vi "Configure FRTD.vi"(0 "VISA resource name":refnum<visa-resource-name>, 1 "FRTD Type (0: PT100)":u16(ring) items=["PT100", "D100", "F100", "PT3916", "PT385", "USER"], 5 "error in (no error)":errorcluster, 6 "Scan List (Empty)":string, 7 "R Zero (100)":i32=100, 9 "Alpha (0.00385)":dbl=0.00385, 11 "Beta (0.111)":dbl=0.111, 13 "Delta (1.507)":dbl=1.507) -> (14 "VISA resource name out":refnum<visa-resource-name>, 19 "error out":errorcluster)   [LabVIEW 2020, in "Keithley 27XX.lvlib"]
doc: "This VI sets the transducer type to 4-wire RTD. It also provided for configuration of a 4-wire RTD measurement.\n\nNote: \n(1) Configure Measurement.vi must be called <B>before</B> running this VI.\n\n(2) This VI will only work if the DMM is in Temperature Measurement mode.\n\n(3) The temperature measurement range for 4-wire RTDs is -200 to 630 deg C (0.001 deg C resolution)\n\n(4) Temperature is calculated using Callendar-Van Dusen equation.\n\n(5) The RTD has a metal construction (typically platinum). The resistance of the RTD changes with change in temperature. The DMM measures teh resistance and calculates the temperature reading. When using default RTD parameters, the resistance of the RTD will be 100 ohms at 0 deg.\n\n(6) Of all the temperature transducers, the RTD exhibits the most stability and linearity. The DMM performs the 4-wire measurement using offset-compensated ohms. This provides the most accurate way to measure the low resistance of the RTD."
uses:
  <instrlib>/Keithley 27XX/Keithley 27XX.lvlib
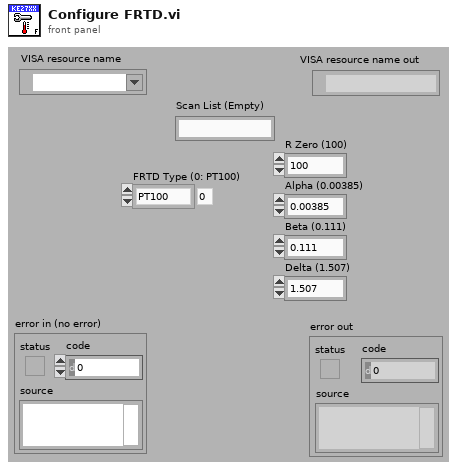
[diagram p1: front panel]
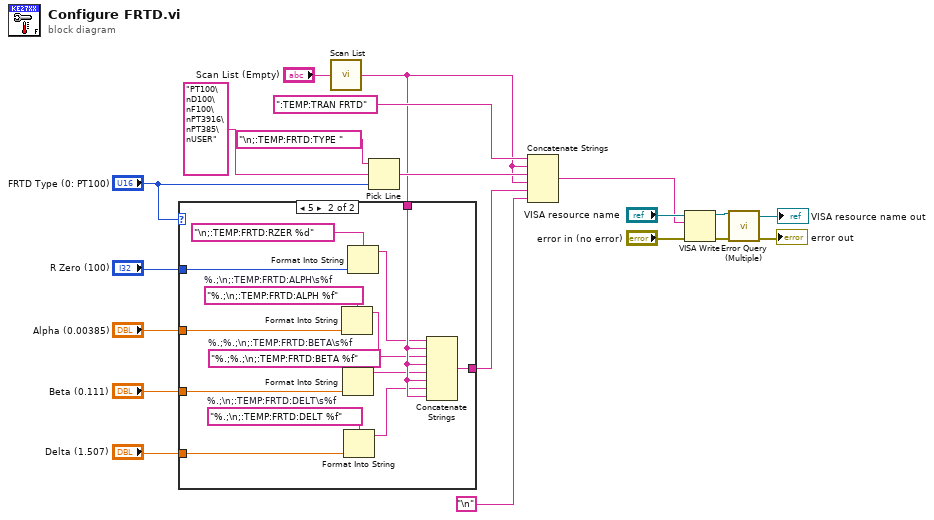
[diagram p0: block diagram]
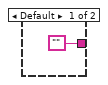
[diagram p2: hidden frame]
diagram:
  n1 = call <instrlib>:"Scan List.vi"("Scan List (Empty)"="Scan List (Empty)") -> ("Scan List Out"=w6:string)  [unwired: 14 in]
  n2 = case shown="5" "FRTD Type (0: PT100)" {
    tunnel: "R Zero (100)" -> [_ w32]
    tunnel: "Alpha (0.00385)" -> [_ w29]
    tunnel: "Beta (0.111)" -> [_ w26]
    tunnel: "Delta (1.507)" -> [_ w23]
    tunnel: ["" w35] -> w13
    tunnel: w6 -> [_ w34]
    frame Default {
    }
    frame 5 {
      w24 = "%.;\n;:TEMP:FRTD:DELT %f"  # %.;\n;:TEMP:FRTD:DELT\s%f
      w27 = "%.;%.;\n;:TEMP:FRTD:BETA %f"  # %.;%.;\n;:TEMP:FRTD:BETA\s%f
      w30 = "%.;\n;:TEMP:FRTD:ALPH %f"  # %.;\n;:TEMP:FRTD:ALPH\s%f
      n3 = Format Into String(format string=w30, w29) -> (resulting string=w28:string)  [unwired: 2 in, 1 out]
      n4 = Format Into String(format string=w27, w26) -> (resulting string=w25:string)  [unwired: 2 in, 1 out]
      n5 = Format Into String(format string=w24, w23) -> (resulting string=w22:string)  [unwired: 2 in, 1 out]
      n6 = Format Into String(format string="\n;:TEMP:FRTD:RZER %d", w32) -> (resulting string=w31:string)  [unwired: 2 in, 1 out]
      n7 = Concatenate Strings(w31, w34, w28, w34, w25, w34, w22, w34) -> (w35:string)
    }
  }
  n8 = Pick Line(string ("")="\n;:TEMP:FRTD:TYPE ", multi-line string="PT100\nD100\nF100\nPT3916\nPT385\nUSER", line index="FRTD Type (0: PT100)") -> (output string=w7:string)
  n9 = Concatenate Strings(":TEMP:TRAN FRTD", w6, w7, w6, w13, "\n") -> (w10:string)
  n10 = VISA Write(VISA resource name="VISA resource name", write buffer=w10, error in (no error)="error in (no error)") -> (VISA resource name out=w5:refnum<visa-resource-name>, error out=w4:errorcluster)  [unwired: 1 out]
  n11 = call <instrlib>:"Error Query (Multiple).vi"("VISA resource name"=w5, "error in (no error)"=w4) -> ("VISA resource name out"=→"VISA resource name out":refnum<visa-resource-name>, "error out"=→"error out":errorcluster)  [unwired: 10 in, 2 out]
